vi "StageToPos.vi"(8 "error in (no error)":errorcluster, 9 "Move to pos":dbl, 10 "Stage Select":T1, 11 "Device In":T2) -> (0 "error out":errorcluster)   [LabVIEW 2014]
doc: "Move the stage to an absolute position"
uses:
  C:/Users/light/Desktop/SI+Raman/Labview/Raman/dll/ThorLabs.MotionControl.KCube.DCServoCLI.dll
  dll/ThorLabs.MotionControl.KCube.DCServoCLI.dll
  TypeDef/StageDeviceOut.ctl
  TypeDef/StageSelect.ctl
panel:
  # "Move the stage to an absolute position"
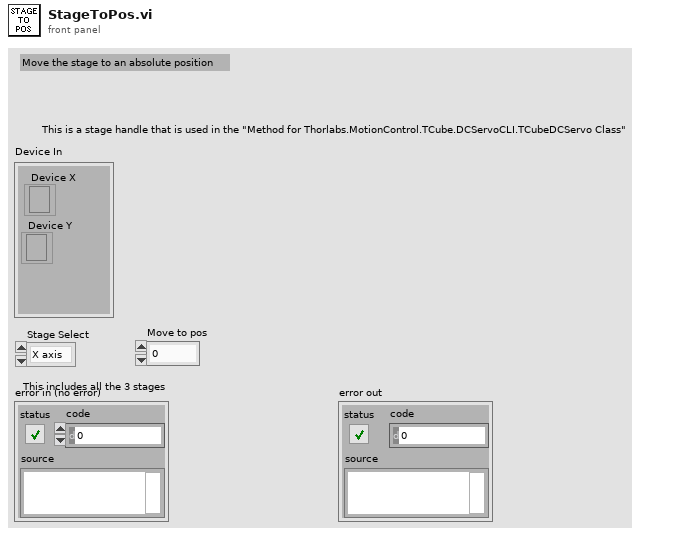
[diagram p1: front panel]
types:
  T1 = typedef "StageSelect.ctl" = enum16{"X axis", "Y axis", "Z axis"}
  T2 = typedef "StageDeviceOut.ctl" = cluster{"Device X":refnum<k24>, "Device Y":refnum<k24>}
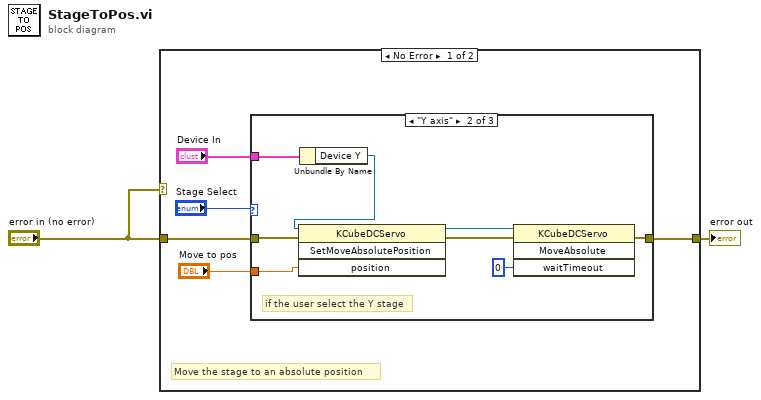
[diagram p0: block diagram]
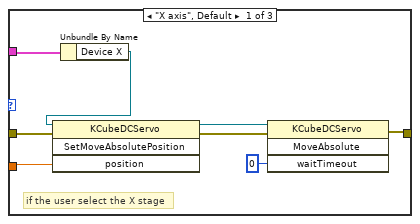
[diagram p2: hidden frame]
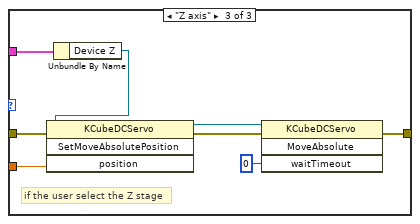
[diagram p3: hidden frame]
diagram:
  n1 = case shown="No Error" "error in (no error)" {
    tunnel: "error in (no error)" -> [w7 w32]
    tunnel: [w5 w32] -> w1
    frame No Error {
      # "Move the stage to an absolute position"
      n2 = case shown="\"Y axis\"" "Stage Select" {
        tunnel: w7 -> [w10 w17 w29]
        tunnel: [w8 w20 w27] -> w5
        tunnel: "Device In" -> [w15 w23 w30]
        tunnel: "Move to pos" -> [w9 w16 w25]
        frame "X axis", Default {
          # "if the user select the X stage"
          n3 = Unbundle By Name(w15) -> ("Device X"=w11:refnum<k24>)
          n4 = invoke class="KCubeDCServo" method="SetMoveAbsolutePosition"(reference=w11, error in=w10, "position"=w9) -> (reference out=w12:refnum<k24>, error out=w13:errorcluster)  [unwired: 1 in, 2 out]
          n5 = invoke class="KCubeDCServo" method="MoveAbsolute"(reference=w12, error in=w13, "waitTimeout"=0) -> (error out=w8:errorcluster)  [unwired: 1 in, 3 out]
        }
        frame "Y axis" {
          # "if the user select the Y stage"
          n6 = Unbundle By Name(w23) -> ("Device Y"=w18:refnum<k24>)
          n7 = invoke class="KCubeDCServo" method="SetMoveAbsolutePosition"(reference=w18, error in=w17, "position"=w16) -> (reference out=w19:refnum<k24>, error out=w22:errorcluster)  [unwired: 1 in, 2 out]
          n8 = invoke class="KCubeDCServo" method="MoveAbsolute"(reference=w19, error in=w22, "waitTimeout"=0) -> (error out=w20:errorcluster)  [unwired: 1 in, 3 out]
        }
        frame "Z axis" {
          # "if the user select the Z stage"
          n9 = Unbundle By Name(w30) -> ("Device Z"=w31:refnum<k24>)
          n10 = invoke class="KCubeDCServo" method="SetMoveAbsolutePosition"(reference=w31, error in=w29, "position"=w25) -> (reference out=w24:refnum<k24>, error out=w28:errorcluster)  [unwired: 1 in, 2 out]
          n11 = invoke class="KCubeDCServo" method="MoveAbsolute"(reference=w24, error in=w28, "waitTimeout"=0) -> (error out=w27:errorcluster)  [unwired: 1 in, 3 out]
        }
      }
    }
    frame Error {
    }
  }
  "error out" <- w1
